vi "IR_READ_WRITE.vi"(5 "Excel Sheet Name":string, 7 "Peak Heights(comma separated)":string, 8 "error constant":errorcluster, 9 "Number of files to read":dbl=1.0, 10 "Report temp":string, 11 "IR Read Dir.":string) -> (0 "error constant 2":errorcluster, 2 "averagePeaksStr":string, 3 "averagePeaks":dbl[](array[numeric]), 4 "Is SS?":bool)   [LabVIEW 2015]
panel:
  in  "XL Sheet Name":string
  in  "Report File":string
  # "IR Data Read and Write"
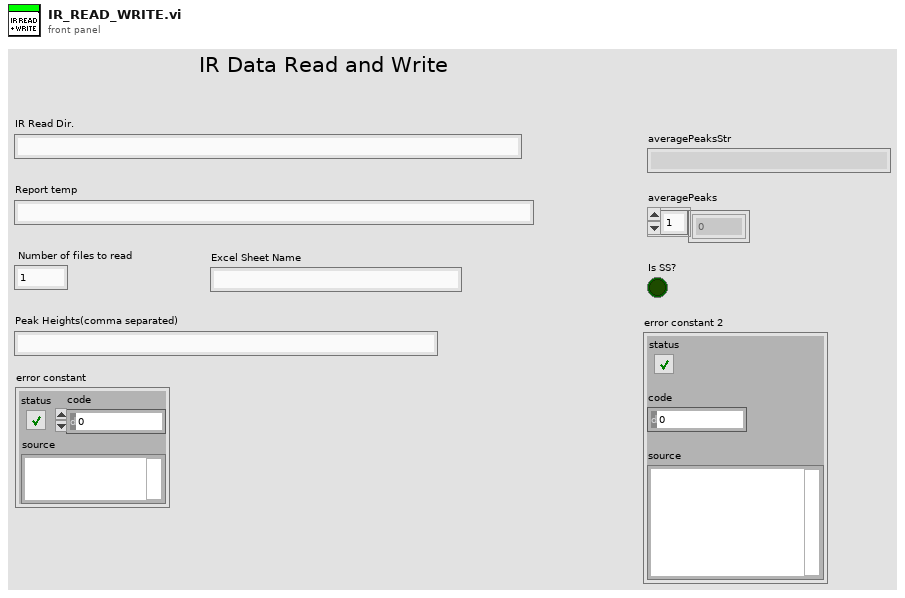
[diagram p1: front panel]
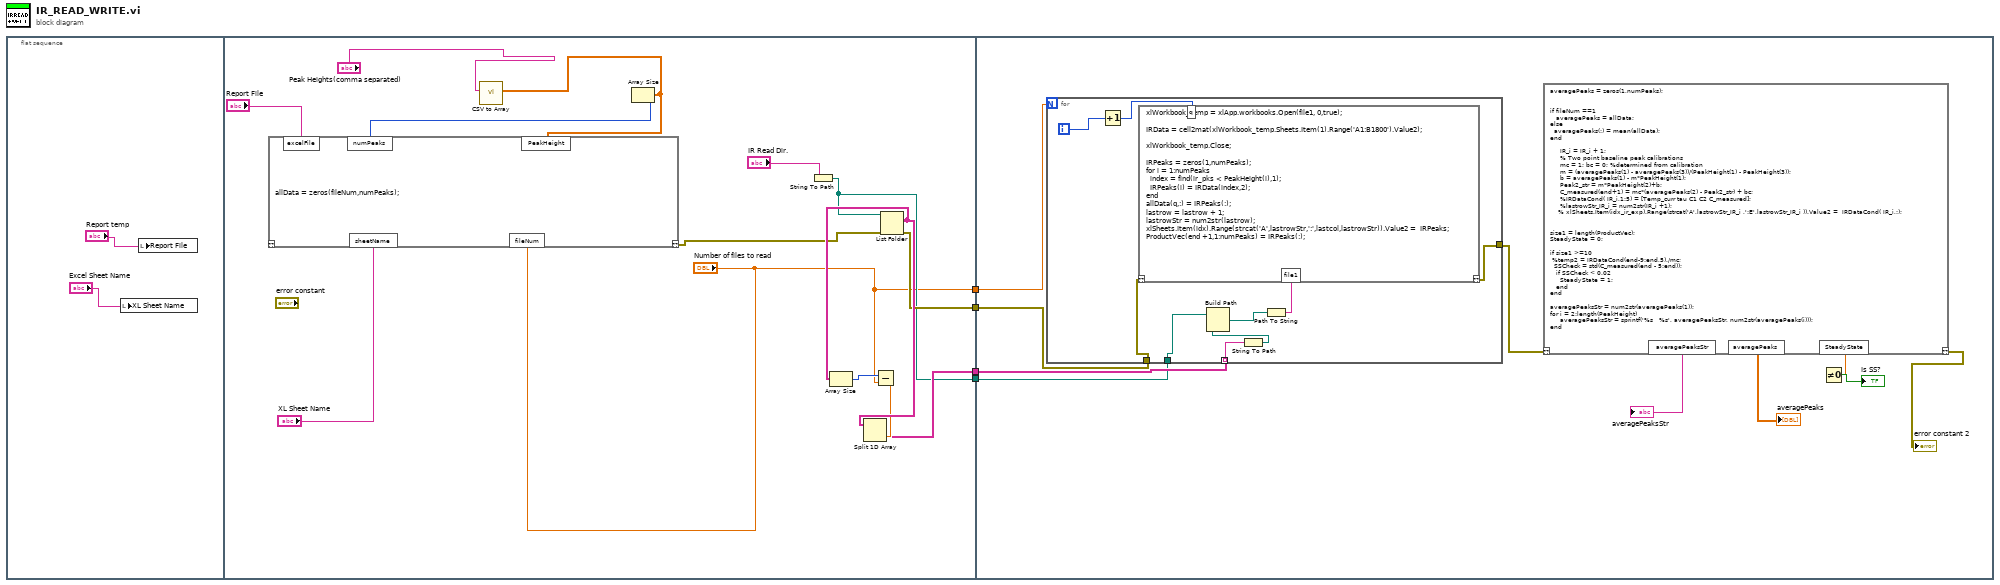
[diagram p0: block diagram]
diagram:
  n1 = flat-sequence {
    tunnel: [w12] -> w4
    tunnel: [w11] -> w3
    tunnel: [w10] -> w2
    tunnel: ["Number of files to read"] -> w1
    tunnel: w4 -> [w24]
    tunnel: w3 -> [w23]
    tunnel: w2 -> [w22]
    tunnel: w1 -> [w21]
    frame #0 {
      n2 = local write "XL Sheet Name"("Excel Sheet Name") -> ()
      n3 = local write "Report File"("Report temp") -> ()
    }
    frame #1 {
      n4 = call "CSV to Array.vi"("Comma Separated floating point number"="Peak Heights(comma separated)") -> ("output array"=w7:dbl[])  [unwired: 10 in]
      n5 = Array Size(array=w7) -> (size(s)=w14:i32)
      n6 = script code="allData = zeros(fileNum,numPeaks);"("numPeaks"=w14, "PeakHeight"=w7, "excelFile"="Report File", "sheetName"="XL Sheet Name", "fileNum"="Number of files to read") -> ("??"=w13:errorcluster)  [unwired: 1 in]
      n7 = String To Path(string="IR Read Dir.") -> (path=w10:path)
      n8 = List Folder(path=w10, error in=w13) -> (filenames=w18:string[], error out=w12:errorcluster)  [unwired: 2 in, 2 out]
      n9 = Array Size(array=w18) -> (size(s)=w16:i32)
      n10 = Subtract(x=w16, y="Number of files to read") -> (x-y=w17:dbl)
      n11 = Split 1D Array(array=w18, index=w17) -> (second subarray=w11:string[])  [unwired: 1 out]
    }
    frame #2 {
      n12 = for {
        N: w21 -> [_]
        tunnel: w22 -> [w39]
        tunnel: w23 -> [w38] mode=indexing
        tunnel: [w33] -> w25
        tunnel: w24 -> [w32]
        i -> [w35]
        n13 = Increment(x=w35) -> (x+1=w34:i32)
        n14 = String To Path(string=w38) -> (path=w37:path)
        n15 = Build Path(base path=w39, name or relative path=w37) -> (appended path=w36:path)
        n16 = Path To String(path=w36) -> (string=w31:string)
        n17 = script code="xlWorkbook_temp = xlApp.workbooks.Open(file1, 0,true);\n\nIRData = cell2mat(xlWorkbook_temp.Sheets.Item(1).Range('A1:B1800').Value2); \n\nxlWorkbook_temp.Close;\n\nIRPeaks = zeros(1,numPeaks);\nfor i = 1:numPeaks\n  index = find(ir_pks < PeakHeight(i),1);\n  IRPeaks(i) = IRData(index,2);\nend\nallData(q,:) = IRPeaks(:);\nlastrow = lastrow + 1;\nlastrowStr = num2str(lastrow);\nxlSheets.Item(idx).Range(strcat('A',lastrowStr,':',lastcol,lastrowStr)).Value2 =  IRPeaks;\nProductVec(end +1,1:numPeaks) = IRPeaks(:);"("??"=w32, "q"=w34, "file1"=w31) -> ("??"=w33:errorcluster)
      }
      n18 = script code="averagePeaks = zeros(1,numPeaks);\n\n\nif fileNum ==1 \n   averagePeaks = allData;\nelse\n  averagePeaks(:) = mean(allData);\nend\n\n     IR_i = IR_i + 1;\n     % Two point baseline peak calibrations\n     mc = 1; bc = 0; %determined from calibration\n     m = (averagePeaks(1) - averagePeaks(3))/(PeakHeight(1) - PeakHeight(3));\n     b = averagePeaks(1) - m*PeakHeight(1);\n     Peak2_str = m*PeakHeight(2)+b;\n     C_measured(end+1) = mc*(averagePeaks(2) - Peak2_str) + bc;\n     %IRDataCond( IR_i,1:5) = [Temp_curr tau C1 C2 C_measured];\n     %lastrowStr_IR_i = num2str(IR_i +1);\n    % xlSheets.Item(idx_ir_exp).Range(strcat('A',lastrowStr_IR_i ,':E',lastrowStr_IR_i )).Value2 =  IRDataCond( IR_i,:);\n\n\nsize1 = length(ProductVec);\nSteadyState = 0;\n\nif size1 >=10\n %temp2 = IRDataCond(end-9:end,5)./mc;\n  SSCheck = std(C_measured(end - 5:end));\n   if SSCheck < 0.02\n     SteadyState = 1;\n   end\nend\n\naveragePeaksStr = num2str(averagePeaks(1));\nfor i = 2:length(PeakHeight)\n     averagePeaksStr = sprintf('%s   %s', averagePeaksStr, num2str(averagePeaks(i)));\nend"("??"=w25) -> ("??"=→"error constant 2":errorcluster, "SteadyState"=w27:dbl, "averagePeaksStr"=→"averagePeaksStr":string, "averagePeaks"=→"averagePeaks":dbl[])
      n19 = Not Equal To 0?(x=w27) -> (x != 0?=→"Is SS?":bool)
    }
  }
